vi "Make Templates From Snips.vi"() -> ()   [LabVIEW 2015]
panel:
  out "error out":errorcluster
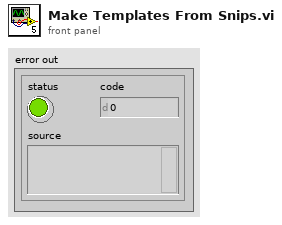
[diagram p1: front panel]
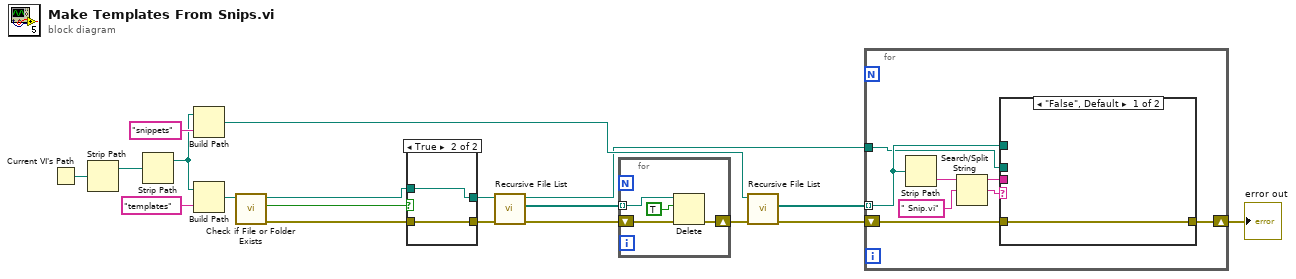
[diagram p0: block diagram]
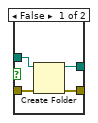
[diagram p2: hidden frame]
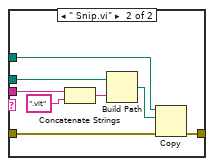
[diagram p3: hidden frame]
diagram:
  n1 = Current VI's Path() -> (path=w19:path)
  n2 = Strip Path(path=w19) -> (stripped path=w18:path)  [unwired: 1 out]
  n3 = Strip Path(path=w18) -> (stripped path=w13:path)  [unwired: 1 out]
  n4 = Build Path(base path=w13, name or relative path="snippets") -> (appended path=w16:path)
  n5 = Build Path(base path=w13, name or relative path="templates") -> (appended path=w5:path)
  n6 = call <vilib>:"Check if File or Folder Exists.vi"("path"=w5) -> ("error out"=w3:errorcluster, "file or folder exists?"=w2:bool, "dup path"=w4:path)  [unwired: 8 in]
  n7 = case shown="True" w2 {
    tunnel: [w23 w24] -> w11
    tunnel: [w22 w25] -> w10
    tunnel: w4 -> [w21 w24]
    tunnel: w3 -> [w20 w25]
    frame False {
      n8 = Create Folder(path (use dialog)=w21, error in=w20) -> (created path=w23:path, error out=w22:errorcluster)  [unwired: 1 in, 1 out]
    }
    frame True {
    }
  }
  n9 = call <vilib>:"Recursive File List.vi"("error in (no error)"=w10, "Folder Path"=w11) -> ("error out"=w9:errorcluster, "All Files in Dir"=w12:path[], "dup Folder Path"=w1:path)  [unwired: 5 in, 2 out]
  n10 = for {
    tunnel: w12 -> [w28] mode=indexing
    shift-right: [w26] -> w8
    shift-left: w9 -> [w27]
    n11 = Delete(path (use dialog)=w28, entire hierarchy (F)=TRUE, error in=w27) -> (error out=w26:errorcluster)  [unwired: 2 in, 2 out]
  }
  n12 = call <vilib>:"Recursive File List.vi"("error in (no error)"=w8, "Folder Path"=w16) -> ("error out"=w7:errorcluster, "All Files in Dir"=w15:path[])  [unwired: 5 in, 3 out]
  n13 = for {
    tunnel: w15 -> [w34] mode=indexing
    shift-right: [w32] -> w6
    shift-left: w7 -> [w33]
    tunnel: w1 -> [w31]
    n14 = Strip Path(path=w34) -> (name=w37:string)  [unwired: 1 out]
    n15 = Search/Split String(string=w37, search string/char (-)=" Snip.vi") -> (substring before match=w35:string, match + rest of string=w30:string)  [unwired: 1 in, 1 out]
    n16 = case shown="\"False\", Default" w30 {
      tunnel: w35 -> [_ w46]
      tunnel: w34 -> [_ w43]
      tunnel: w33 -> [w38 w41]
      tunnel: [w38 w40] -> w32
      tunnel: w31 -> [_ w39]
      frame "False", Default {
      }
      frame " Snip.vi" {
        n17 = Concatenate Strings(w46, ".vit" ("string")) -> (w44:string)
        n18 = Build Path(base path=w39, name or relative path=w44) -> (appended path=w42:path)
        n19 = Copy(8:w41, 10:w42, 11:w43) -> (0:w40:errorcluster)  [unwired: 2 in, 2 out]
      }
    }
  }
  "error out" <- w6
